vi "oa_Get 3 Stage Half Band Interpolation Filter Coefficients.vi"(7 "reset? (True)":bool=TRUE, 11 "A stop [dB]":dbl=120.0) -> (1 "interpolation filter info":cluster{i32, "y":i32}[](array[cluster]), 3 "interpolation filters":T1[](array[typedef]) {"coefficients" format="%.2f"})   [LabVIEW 2017, in "SoundVib_Resampling.lvlib"]
uses:
  <vilib>/addons/Sound and Vibration/Order Analysis/Resample Order Tracking/SoundVib_Resampling.lvlib
  <vilib>/addons/_NISVFA/_Shared subVIs/Controls/OAT Decimation Filter.ctl
panel:
  in  "Case Constant\n(See Context Help)":bool=TRUE
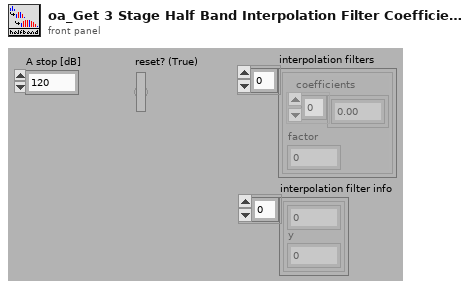
[diagram p1: front panel]
types:
  T1 = typedef "OAT Decimation Filter.ctl" = cluster{"coefficients":dbl[], "factor":i32}
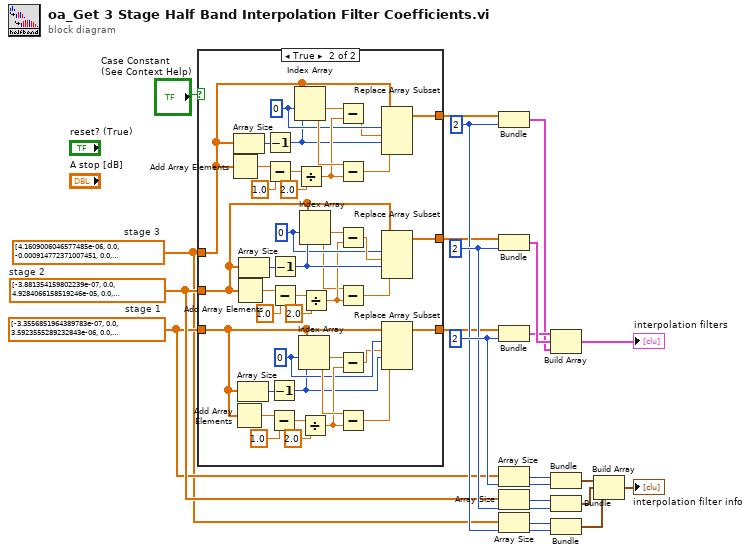
[diagram p0: block diagram]
diagram:
  w4 = dbl[] [4.1609006046577485e-06, 0.0, -0.000914772371007451, 0.0, 0.01067071711716509, 0.0, -0.05775967594558672, 0.0, 0.29800126331908455, 0.5, 0.29800126331908455, 0.0, -0.05775967594558672, 0.0, 0.01067071711716509, 0.0, -0.000914772371007451, 0.0, 4.1609006046577485e-06]  # stage 3
  w6 = dbl[] [-3.881354159802239e-07, 0.0, 4.9284066158519246e-05, 0.0, -0.0005314545848909713, 0.0, 0.0028836957885210136, 0.0, -0.010648565187532658, 0.0, 0.031006551310363683, 0.0, -0.08227486341490464, 0.0, 0.30951554176898005, 0.5, 0.30951554176898005, 0.0, -0.08227486341490464, 0.0, 0.031006551310363683, 0.0, -0.010648565187532658, 0.0, 0.0028836957885210136, 0.0, -0.0005314545848909713, 0.0, 4.9284066158519246e-05, 0.0, -3.881354159802239e-07]  # stage 2
  w5 = dbl[] [-3.3556851964389783e-07, 0.0, 3.5923555289232843e-06, 0.0, -1.4701244639626162e-05, 0.0, 4.34993136449147e-05, 0.0, -0.0001070096574468051, 0.0, 0.00023222057920717484, 0.0, -0.0004590438459981563, 0.0, 0.0008432595824871062, 0.0, -0.0014593782710335128, 0.0, 0.0024036743506056285, 0.0, -0.00379830435761134, 0.0, 0.005798695595796536, 0.0, -0.008608969490996472, 0.0, 0.012515943559406778, 0.0, -0.017967010357116734, 0.0, 0.025760935970907912, 0.0, -0.03757643886042131, 0.0, 0.057780126171606404, 0.0, -0.10247327868967936, 0.0, 0.3170826192030624, 0.5, 0.3170826192030624, 0.0, -0.10247327868967936, 0.0, 0.057780126171606404, 0.0, -0.03757643886042131, 0.0, 0.025760935970907912, 0.0, -0.017967010357116734, 0.0, 0.012515943559406778, 0.0, -0.008608969490996472, 0.0, 0.005798695595796536, 0.0, -0.00379830435761134, 0.0, 0.0024036743506056285, 0.0, -0.0014593782710335128, 0.0, 0.0008432595824871062, 0.0, -0.0004590438459981563, 0.0, 0.00023222057920717484, 0.0, -0.0001070096574468051, 0.0, 4.34993136449147e-05, 0.0, -1.4701244639626162e-05, 0.0, 3.5923555289232843e-06, 0.0, -3.3556851964389783e-07]  # stage 1
  w17 = 2 ("y")
  w15 = 2 ("y")
  w13 = 2 ("y")
  n1 = case shown="True" "Case Constant\n(See Context Help)" {
    tunnel: w4 -> [w22 w58]
    tunnel: [w22 w53] -> w3
    tunnel: w6 -> [w24 w40]
    tunnel: [w24 w39] -> w8
    tunnel: w5 -> [w23 w26]
    tunnel: [w23 w25] -> w7
    frame False {
    }
    frame True {
      w30 = 0 ("index")
      w49 = 0 ("index")
      w57 = 0 ("index")
      n2 = Add Array Elements(numeric array=w58) -> (sum=w66:dbl)
      n3 = Array Size(array=w58) -> (size(s)=w62:i32)
      n4 = Add Array Elements(numeric array=w26) -> (sum=w38:dbl)
      n5 = Add Array Elements(numeric array=w40) -> (sum=w41:dbl)
      n6 = Array Size(array=w26) -> (size(s)=w34:i32)
      n7 = Array Size(array=w40) -> (size(s)=w45:i32)
      n8 = Decrement(x=w62) -> (x-1=w55:i32)
      n9 = Subtract(x=w66, y=1.0) -> (x-y=w64:dbl)
      n10 = Decrement(x=w34) -> (x-1=w28:i32)
      n11 = Subtract(x=w38, y=1.0) -> (x-y=w36:dbl)
      n12 = Decrement(x=w45) -> (x-1=w51:i32)
      n13 = Subtract(x=w41, y=1.0) -> (x-y=w43:dbl)
      n14 = Index Array(array=w58, index #1=w57, index #2=w55) -> (element #1=w61:dbl, element #2=w60:dbl)
      n15 = Divide(x=w64, y=2.0) -> (x/y=w59:dbl)
      n16 = Index Array(array=w26, index #1=w30, index #2=w28) -> (element #1=w33:dbl, element #2=w32:dbl)
      n17 = Index Array(array=w40, index #1=w49, index #2=w51) -> (element #1=w46:dbl, element #2=w47:dbl)
      n18 = Divide(x=w36, y=2.0) -> (x/y=w31:dbl)
      n19 = Divide(x=w43, y=2.0) -> (x/y=w48:dbl)
      n20 = Subtract(x=w61, y=w59) -> (x-y=w56:dbl)
      n21 = Subtract(x=w60, y=w59) -> (x-y=w54:dbl)
      n22 = Subtract(x=w46, y=w48) -> (x-y=w50:dbl)
      n23 = Subtract(x=w47, y=w48) -> (x-y=w52:dbl)
      n24 = Subtract(x=w33, y=w31) -> (x-y=w29:dbl)
      n25 = Subtract(x=w32, y=w31) -> (x-y=w27:dbl)
      n26 = Replace Array Subset(array=w58, new element #1=w56, index #1=w57, new element #2=w54, index #2=w55) -> (w53:dbl[])
      n27 = Replace Array Subset(array=w40, new element #1=w50, index #1=w49, new element #2=w52, index #2=w51) -> (w39:dbl[])
      n28 = Replace Array Subset(array=w26, new element #1=w29, index #1=w30, new element #2=w27, index #2=w28) -> (w25:dbl[])
    }
  }
  n29 = Bundle("stage 3"=w3, "y"=w13) -> (w2:cluster{"stage 3":dbl[], "y":i32})  [unwired: 1 in]
  n30 = Bundle("stage 2"=w8, "y"=w15) -> (w21:cluster{"stage 2":dbl[], "y":i32})  [unwired: 1 in]
  n31 = Bundle("stage 1"=w7, "y"=w17) -> (w20:cluster{"stage 1":dbl[], "y":i32})  [unwired: 1 in]
  n32 = Array Size(array=w5) -> (size(s)=w18:i32)
  n33 = Array Size(array=w6) -> (size(s)=w16:i32)
  n34 = Array Size(array=w4) -> (size(s)=w14:i32)
  n35 = Build Array(w20, w21, w2) -> (→"interpolation filters":cluster{"stage 3":dbl[], "y":i32}[])
  n36 = Bundle(w18, "y"=w17) -> (w12:cluster{i32, "y":i32})  [unwired: 1 in]
  n37 = Bundle(w16, "y"=w15) -> (w11:cluster{i32, "y":i32})  [unwired: 1 in]
  n38 = Bundle(w14, "y"=w13) -> (w1:cluster{i32, "y":i32})  [unwired: 1 in]
  n39 = Build Array(w12, w11, w1) -> (→"interpolation filter info":cluster{i32, "y":i32}[])
